vi "retrieve_device_info.vi"(0 "device_index (in) [0=def]":i32, 5 "Error In":errorcluster) -> (19 "Error Out":errorcluster)   [LabVIEW 2013, in "examples.lvlib"]
doc: "Retrieve the referenced device's information. This example demonstrates the usage of \"member accessors\" which are parameters that were retrieved at device initialization and stored in the Controller class object for later use.\n\nProduced By:\n\n<B>Kod Integrations, LLC</B>\n4835 Marianne Drive\nMount Airy, MD 21771\nhttp://www.kodintegrations.com\nemail: info@kodintegrations.com\nphone: (240) 687-1288"
uses:
  libraries/examples.lvlib
  classes/Controller/_Controller.lvclass
  common/controls/models.ctl
  libraries/common.lvlib
panel:
  out "deviceDesc":string
  out "model":T1
  out "deviceName":string
  out "index":i32
  in  "clear_buffer? (T)":bool=TRUE
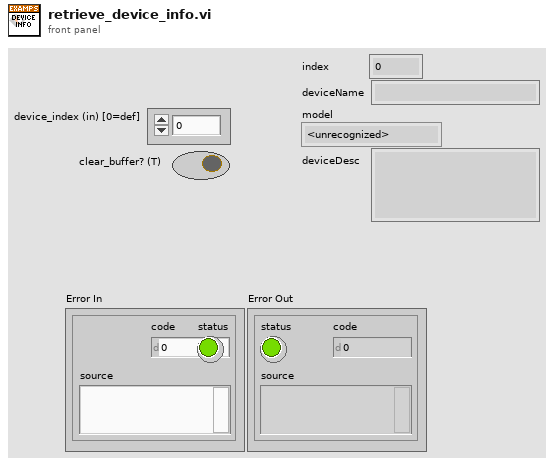
[diagram p1: front panel]
types:
  T1 = typedef "common.lvlib/models.ctl" = enum16{"<unrecognized>", "ACE-SDC", "ACE-SDE", "ACE-SXC", "ACE-SXE", "DMX-CAN", "DMX-J-SA", "DMX-K-SA", "DMX-UMD", "PMX-2ED-SA", "PMX-2EX-SA", "PMX-4CX-SA", "PMX-4EX-SA"}
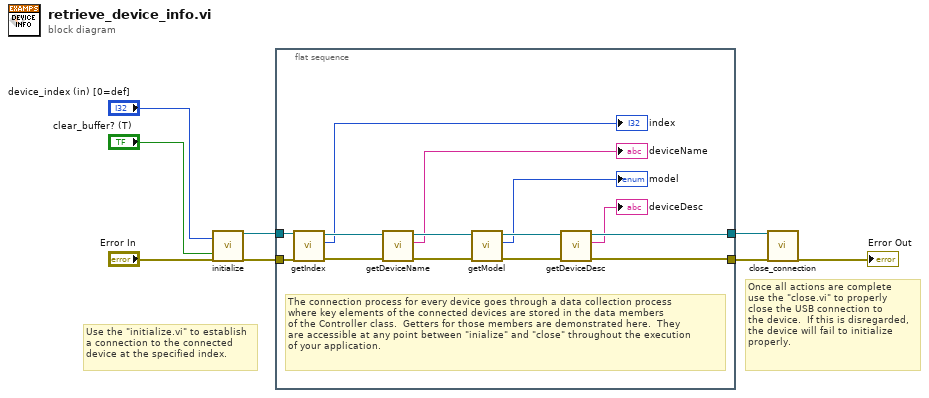
[diagram p0: block diagram]
diagram:
  # "Once all actions are complete\nuse the \"close.vi\" to properly\nclose the USB connection to \nthe device.  If this is disregarded,\nthe device will fail to initialize \nproperly."
  # "Use the \"initialize.vi\" to establish\na connection to the connected\ndevice at the specified index."
  n1 = call "initialize.vi"("device_index (in) [0=def]"="device_index (in) [0=def]", "clear_buffer? (T)"="clear_buffer? (T)", "error in (no error)"="Error In") -> ("reference (out)"=w5:refnum<class "_Controller.lvclass">, "error out"=w4:errorcluster)  [unwired: 15 in]
  n2 = flat-sequence {
    tunnel: w5 -> [w22]
    tunnel: w4 -> [w17]
    tunnel: [w18] -> w3
    tunnel: [w13] -> w2
    frame #0 {
      # "The connection process for every device goes through a data collection process\nwhere key elements of the connected devices are stored in the data members\nof the Controller class.  Getters for those members are demonstrated here.  They\nare accessible at any point between \"inialize\" and \"close\" throughout the execution\nof your application."
      n3 = call "getIndex.vi"("error in (no error)"=w17, "reference (in)"=w22) -> ("error out"=w16:errorcluster, "index"=→"index":i32, "reference (out)"=w21:refnum<class "_Controller.lvclass">)  [unwired: 7 in]
      n4 = call "getDeviceName.vi"("error in (no error)"=w16, "reference (in)"=w21) -> ("error out"=w15:errorcluster, "deviceName"=→"deviceName":string, "reference (out)"=w20:refnum<class "_Controller.lvclass">)  [unwired: 7 in]
      n5 = call "getModel.vi"("error in (no error)"=w15, "reference (in)"=w20) -> ("error out"=w14:errorcluster, "model"=→"model":T1, "reference (out)"=w19:refnum<class "_Controller.lvclass">)  [unwired: 7 in]
      n6 = call "getDeviceDesc.vi"("error in (no error)"=w14, "reference (in)"=w19) -> ("error out"=w13:errorcluster, "deviceDesc"=→"deviceDesc":string, "reference (out)"=w18:refnum<class "_Controller.lvclass">)  [unwired: 7 in]
    }
  }
  n7 = call "close_connection.vi"("reference (in)"=w3, "error in (no error)"=w2) -> ("error out"=→"Error Out":errorcluster)  [unwired: 16 in, 1 out]
